vi "Panel.vi"(11 "DoublePanel in":refnum<class "DoublePanel.lvclass">) -> ()   [LabVIEW 2020, in "Conditum-Tools.lvlib" / "DoublePanel.lvclass"]
uses:
  DoublePanel.lvclass
  C:/dev/lv20CE/lv-conditum/Conditum-Tools/ColumnPanel/ColumnPanel.lvclass
  C:/Program Files (x86)/National Instruments/LabVIEW 2020/vi.lib/IlluminatedG/IG OOPanel/OOPanel/Panel/Panel.lvclass
  ColumnPanel/Common Items.ctl
  <vilib>/IlluminatedG/IG OOPanel/OOPanel/Panel/Basic UI State.ctl
  Conditum/Columns/Double/Double.lvclass
  C:/dev/lv20CE/lv-conditum/Conditum/Columns/Type/Type.lvclass
  Conditum/Columns/Type/Type.lvclass/Type.ctl
  DoublePanel.lvclass/DoublePanel.ctl
  Conditum/Columns/Double/Double Definition.ctl
  Conditum/Columns/Type/Definition.ctl
  Conditum/Attributes.ctl
  Conditum/Columns/Double/Definition.ctl
  0a21f17a-76fb-470e-98eb-44d75b556dd5.vi
  Conditum/Columns/Type/Type.lvclass
  <vilib>/IlluminatedG/IG OOPanel/OOPanel/Panel/Panel.lvclass
  ColumnPanel/ColumnPanel.lvclass
  Conditum/Conditum.lvlib
  <vilib>/IlluminatedG/IG OOPanel/OOPanel/OOPanel.lvlib
panel:
  in  "Default Value":dbl
  in  "Common Items":T1
  # "Double"
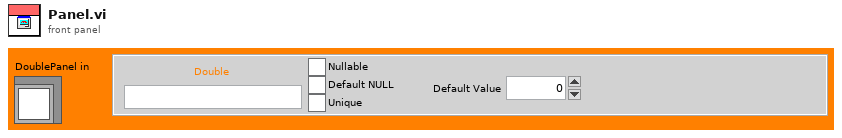
[diagram p1: front panel]
types:
  T1 = typedef "Conditum-Tools.lvlib/ColumnPanel.lvclass/Common Items.ctl" = cluster{"Name":string, "Nullable":bool, "Default NULL":bool, "Unique":bool}
  T2 = typedef "OOPanel.lvlib/Panel.lvclass/Basic UI State.ctl" = enum16{"Init", "Run", "Close"}
  T3 = typedef "Conditum.lvlib/Columns.lvlib/Double.lvclass/Double Definition.ctl" = cluster{"Type":T4, "Attributes":T5, "Double":T6}
  T4 = typedef "Conditum.lvlib/Columns.lvlib/Type.lvclass/Definition.ctl" = cluster{"Name":string, "Nullable":bool, "Default NULL":bool}
  T5 = typedef "Conditum.lvlib/Attributes.ctl" = cluster{"Primary Key":bool, "Unique":bool, "Foreign Key":bool, "Auto Increment":bool}
  T6 = typedef "Conditum.lvlib/Columns.lvlib/Double.lvclass/Definition.ctl" = cluster{"Default":dbl}
  T7 = typedef "OOPanel.lvlib/Panel.lvclass/Panel Events.ctl" = cluster{"Visbility":refnum<user-event>, "Close":refnum<user-event>}
  T8 = typedef "Conditum-Tools.lvlib/ColumnPanel.lvclass/Events.ctl" = cluster{"Update":refnum<user-event>, "Value":refnum<user-event>, "Valid":refnum<user-event>, "Highlight":refnum<user-event>}
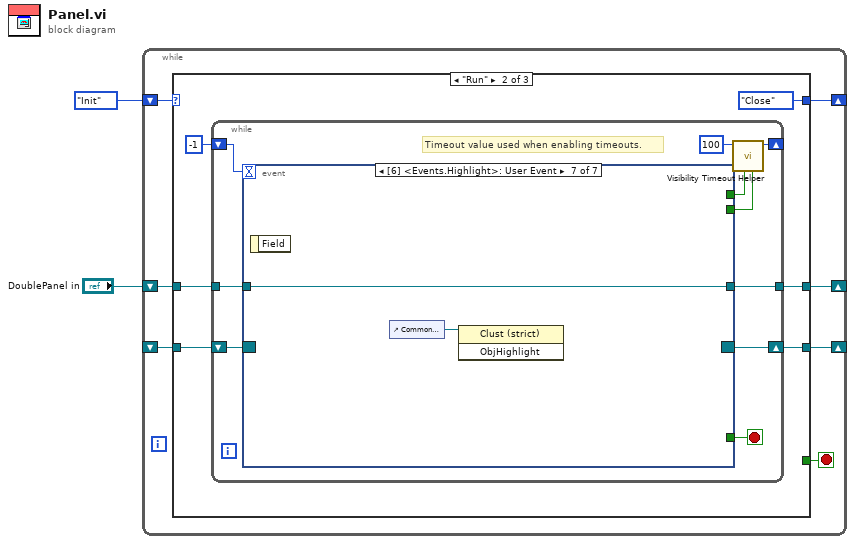
[diagram p0: block diagram]
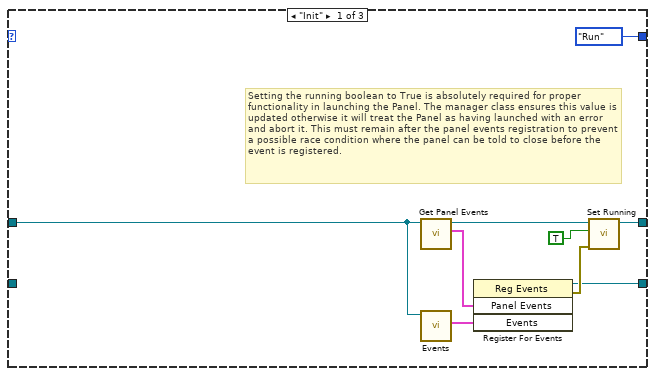
[diagram p2: hidden frame]
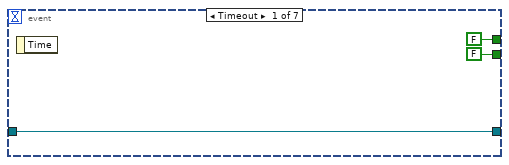
[diagram p3: hidden frame]
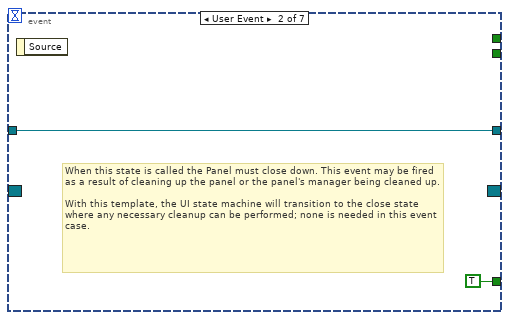
[diagram p4: hidden frame]
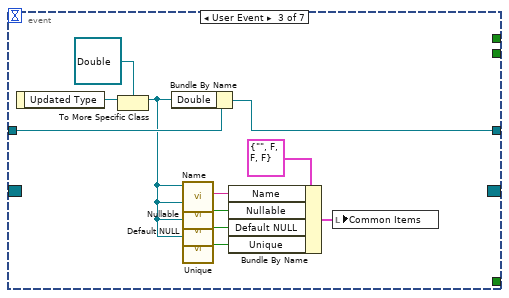
[diagram p5: hidden frame]
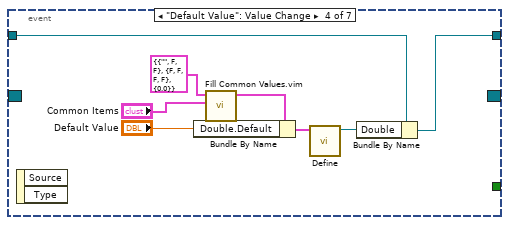
[diagram p6: hidden frame]
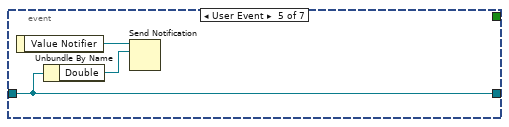
[diagram p7: hidden frame]
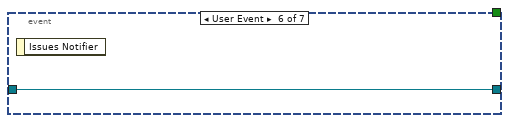
[diagram p8: hidden frame]
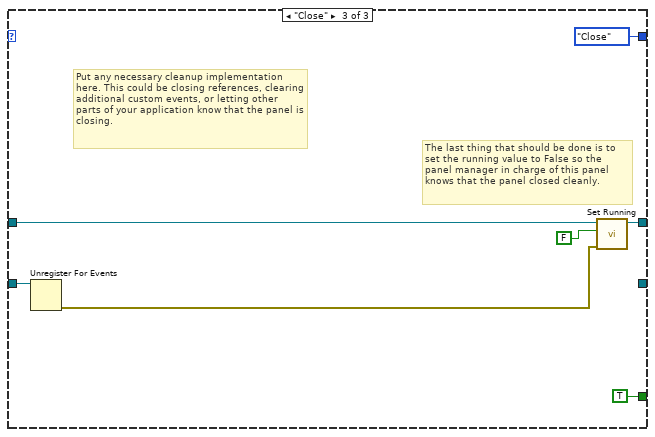
[diagram p9: hidden frame]
diagram:
  n1 = while {
    shift-right: [w8] -> _
    shift-left: _ -> [w9]
    shift-right: [w6] -> _
    shift-left: Basic_UI_State."Init" ("Basic UI State") -> [w7]
    shift-right: [w4] -> _
    shift-left: "DoublePanel in" -> [w3]
    stop <- w5 stop-if-true
    n2 = case shown="\"Run\"" w7 {
      tunnel: w9 -> [_ w24 w67]
      tunnel: [w15 w22 _] -> w8
      tunnel: [Basic_UI_State."Run" ("Basic UI State") Basic_UI_State."Close" ("Basic UI State") Basic_UI_State."Close" ("Basic UI State")] -> w6
      tunnel: [_ _ TRUE] -> w5
      tunnel: [w14 w19 w65] -> w4
      tunnel: w3 -> [w10 w20 w66]
      frame "Init" {
        # "Setting the running boolean to True is absolutely required for proper functionality in launching the Panel. The manager class ensures this value is updated otherwise it will treat the Panel as having launched with an error and abort it. This must remain after the panel events registration to prevent a possible race condition where the panel can be told to close before the event is registered."
        n3 = call <vilib>:"Get Panel Events.vi"("Panel in"=w10) -> ("Panel Events"=w12:T7, "Panel out"=w13:refnum<class "DoublePanel.lvclass">)  [unwired: 8 in, 1 out]
        n4 = call "Events.vi"("ColumnPanel in"=w10) -> ("Events"=w11:T8)  [unwired: 10 in]
        n5 = register-events(w12, w11) -> (reference out=w15:refnum<event-registration>, error out=w17:errorcluster)  [unwired: 2 in]
        n6 = call <vilib>:"Set Running.vi"("error in (no error)"=w17, "Running"=TRUE, "Panel in"=w13) -> ("Panel out"=w14:refnum<class "DoublePanel.lvclass">)  [unwired: 7 in, 1 out]
      }
      frame "Run" {
        n7 = while {
          shift-right: [w30] -> w22
          shift-left: w24 -> [w31]
          shift-right: [w33] -> _
          shift-left: -1 ("Timeout") -> [w32]
          tunnel: w20 -> [w26]
          tunnel: [w25] -> w19
          stop <- w27 stop-if-true
          # "Timeout value used when enabling timeouts."
          n8 = event shown="[6] <Events.Highlight>: User Event" {
            selector: w31 -> [_ _ _ _ _ _ _]
            dyn-events: [_ _ _ _ _ _ _] -> w30
            timeout: w32 -> [_ _ _ _ _ _ _]
            tunnel: [FALSE _ _ _ _ _ _] -> w29
            tunnel: [FALSE _ _ _ _ _ _] -> w28
            tunnel: [_ TRUE _ _ _ _ _] -> w27
            tunnel: w26 -> [w35 w38 w47 w55 w61 w62 w64]
            tunnel: [w35 w38 w48 w56 w61 w62 w64] -> w25
            event Timeout {
              n9 = event-data() -> ()  [unwired: 1 in, 1 out]
            }
            event User Event {
              # "When this state is called the Panel must close down. This event may be fired as a result of cleaning up the panel or the panel's manager being cleaned up.\n\nWith this template, the UI state machine will transition to the close state where any necessary cleanup can be performed; none is needed in this event case."
              n10 = event-data() -> ()  [unwired: 1 in, 1 out]
            }
            event User Event {
              n11 = event-data() -> ("Updated Type"=w50:refnum<class "Type.lvclass">)  [unwired: 1 in]
              n12 = To More Specific Class(target class=refnum<class "Double.lvclass"> refnum ("Conditum:Columns:Double.lvclass"), reference=w50) -> (specific class reference=w40:refnum<class "Double.lvclass">)  [unwired: 1 in, 1 out]
              n13 = Bundle By Name(cluster=w47, "Double"=w40) -> (w48:refnum<class "DoublePanel.lvclass">)
              n14 = call "Name.vi"("Type in"=w40) -> ("Table Name"=w44:string)  [unwired: 10 in]
              n15 = call "Nullable.vi"("Type in"=w40) -> ("Nullable"=w43:bool)  [unwired: 10 in]
              n16 = call "Default NULL.vi"("Type in"=w40) -> ("Default NULL"=w42:bool)  [unwired: 10 in]
              n17 = call "Unique.vi"("Type in"=w40) -> ("Unique"=w41:bool)  [unwired: 10 in]
              n18 = Bundle By Name(cluster=T1 {"Name"="", "Nullable"=FALSE, "Default NULL"=FALSE, "Unique"=FALSE} ("Common Items"), "Name"=w44, "Nullable"=w43, "Default NULL"=w42, "Unique"=w41) -> (w45:T1)
              n19 = local write "Common Items"(w45) -> ()
            }
            event "Default Value": Value Change {
              n20 = event-data() -> ()  [unwired: 1 in, 2 out]
              n21 = call "Fill Common Values.vim"("Common Items"="Common Items", "Init Data Type"=T3 {"Type"={"Name"="", "Nullable"=FALSE, "Default NULL"=FALSE}, "Attributes"={"Primary Key"=FALSE, "Unique"=FALSE, "Foreign Key"=FALSE, "Auto Increment"=FALSE}, "Double"={"Default"=0.0}} ("Init Data")) -> ("Init Data"=w53:T3)  [unwired: 9 in]
              n22 = Bundle By Name(cluster=w53, "Double.Default"="Default Value") -> (w58:T3)
              n23 = call "Define.vi"("Double Definition"=w58) -> ("Double out"=w57:refnum<class "Double.lvclass">)  [unwired: 10 in]
              n24 = Bundle By Name(cluster=w55, "Double"=w57) -> (w56:refnum<class "DoublePanel.lvclass">)
            }
            event User Event {
              n25 = event-data() -> ("Value Notifier"=w60:refnum<notifier>)  [unwired: 1 in]
              n26 = Unbundle By Name(w61) -> ("Double"=w59:refnum<class "Double.lvclass">)
              n27 = Send Notification(notification=w59, notifier=w60) -> ()  [unwired: 1 in, 2 out]
            }
            event User Event {
              n28 = event-data() -> ()  [unwired: 1 in, 1 out]
            }
            event User Event {
              n29 = event-data() -> ()  [unwired: 1 in, 1 out]
              n30 = control-ref of="Common Items"() -> (w63:refnum<vi>)
              n31 = invoke class="Clust (strict)" method="ObjHighlight"(reference=w63) -> ()  [unwired: 2 in, 3 out]
            }
          }
          n32 = call <vilib>:"Visibility Timeout Helper.vi"("Update?"=w28, "Use Timeout?"=w29, "Visible Timeout mS"=100) -> ("Timeout"=w33:i32)  [unwired: 8 in]
        }
      }
      frame "Close" {
        # "Put any necessary cleanup implementation here. This could be closing references, clearing additional custom events, or letting other parts of your application know that the panel is closing."
        # "The last thing that should be done is to set the running value to False so the panel manager in charge of this panel knows that the panel closed cleanly."
        n33 = Unregister For Events(event registration refnum=w67) -> (error out=w69:errorcluster)  [unwired: 1 in]
        n34 = call <vilib>:"Set Running.vi"("error in (no error)"=w69, "Running"=FALSE, "Panel in"=w66) -> ("Panel out"=w65:refnum<class "DoublePanel.lvclass">)  [unwired: 7 in, 1 out]
      }
    }
  }
